vi "ReserveNetworkDAQDevice.vi"() -> ()   [LabVIEW 2022 SP3]
panel:
  out "Error Out":errorcluster
  in  "override reservation?":bool
  in  "device in":tag
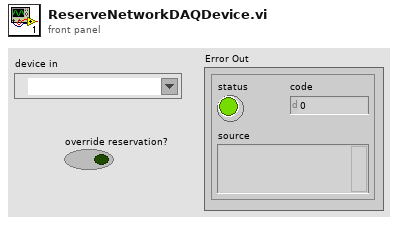
[diagram p1: front panel]
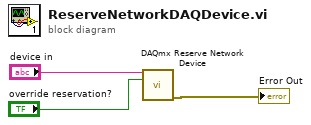
[diagram p0: block diagram]
diagram:
  n1 = call <vilib>:"DAQmx Reserve Network Device.vi"("device in"="device in", "override reservation?"="override reservation?") -> ("error out"=→"Error Out":errorcluster)  [unwired: 12 in, 1 out]
